vi "Write Legend Position.vi"(5 "Legend Position":cluster{"Left":i32, "Top":i32}, 9 "WaveformChart in":refnum<class "WaveformChart.lvclass">) -> (3 "WaveformChart out":refnum<class "WaveformChart.lvclass">)   [LabVIEW 2014, in "WaveformChart.lvclass"]
uses:
  WaveformChart.lvclass
  WaveformChart.lvclass/WaveformChart.ctl
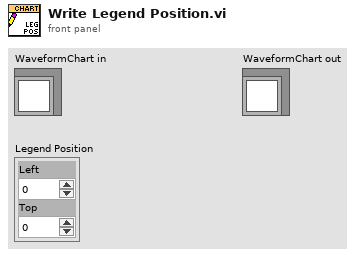
[diagram p1: front panel]
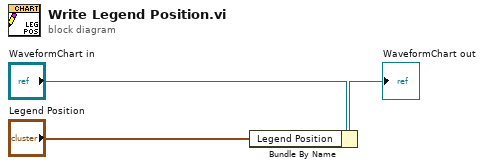
[diagram p0: block diagram]
diagram:
  n1 = Bundle By Name(cluster="WaveformChart in", "Legend Position"="Legend Position") -> (→"WaveformChart out":refnum<class "WaveformChart.lvclass">)
